vi "disk_setTemplateTail.vi"(8 "error in (no error)":errorcluster, 11 "Excel refnum":T1) -> (0 "error out":errorcluster, 2 "template tail":string[](array[string]), 3 "Excel refnum out":T1)   [LabVIEW 2017, in "NI_ExcelFile.lvlib"]
uses:
  <vilib>/express/express shared/NI_ExcelFile/NI_ExcelFile.lvlib
  <vilib>/express/express shared/NI_ExcelFile/Ctrls/ExcelRefnum.ctl
  <vilib>/express/express shared/NI_ExcelFile/Ctrls/MainData.ctl
  <vilib>/express/express shared/NI_ExcelFile/Ctrls/StreamMode.ctl
  <vilib>/express/express shared/NI_ExcelFile/Ctrls/TimeColumnMode.ctl
  <vilib>/express/express shared/NI_ExcelFile/Ctrls/FileAttribute.ctl
  <vilib>/express/express shared/NI_ExcelFile/Ctrls/Columns.ctl
  <vilib>/express/express shared/NI_ExcelFile/Ctrls/ColumnInfo.ctl
  <vilib>/express/express shared/NI_ExcelFile/Ctrls/DataType.ctl
  <vilib>/express/express shared/NI_ExcelFile/Ctrls/wd_recordInfo.ctl
  <vilib>/express/express shared/NI_ExcelFile/Ctrls/disk_TemplateFile.ctl
  <vilib>/express/express shared/NI_ExcelFile/Ctrls/meta_file.ctl
  <vilib>/express/express shared/NI_ExcelFile/Ctrls/meta_Block.ctl
  <vilib>/express/express shared/NI_ExcelFile/Ctrls/meta_BlockType.ctl
  <vilib>/express/express shared/NI_ExcelFile/Ctrls/TemplateEnum.ctl
  <vilib>/express/express shared/NI_ExcelFile/SubVIs/fmt_getUTF-8Text.vi
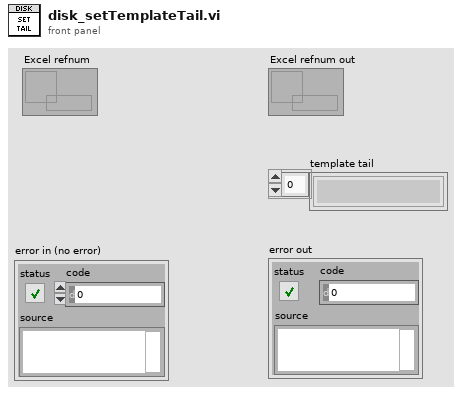
[diagram p1: front panel]
types:
  T1 = typedef "NI_ExcelFile.lvlib/ExcelRefnum.ctl" = refnum<data-value>
  T2 = typedef "NI_ExcelFile.lvlib/MainData.ctl" = cluster{"TargetFile":path, "StreamMode":T3, "Append?":bool, "ChunkSize":u64, "TimeColumnMode":T4, "TimestampFormat":string, "AbsoluteTime?":bool, "FileAttribute ":T5, "Column":T6, "FileRef":refnum<k1>, "MemoryRef":refnum<data-value>[], "RecordInfo":T9[], " ChannelPreviousInfo":u32[], "ChannelFirstRecord":u32[], "PredefinedFormattedValueLength":i64, "DiskTemplate":T10}
  T3 = typedef "NI_ExcelFile.lvlib/StreamMode.ctl" = enum16{"File", "Memory"}
  T4 = typedef "NI_ExcelFile.lvlib/TimeColumnMode.ctl" = enum16{"Empty", "OnePerCh", "One"}
  T5 = typedef "NI_ExcelFile.lvlib/FileAttribute.ctl" = cluster{"Creator":string, "Title":string, "SheetName":string}
  T6 = typedef "NI_ExcelFile.lvlib/Columns.ctl" = T7[]
  T7 = typedef "NI_ExcelFile.lvlib/ColumnInfo.ctl" = cluster{"Header":string, "Format":string, "DataType":T8, "Length":u64}
  T8 = typedef "NI_ExcelFile.lvlib/DataType.ctl" = enum16{"DDT", "WFM", "Array of STR", "Array of DBL", "Array of I8", "Array of I16", "Array of I32", "Array of I64", "Array of SGL", "Array of U8", "Array of U16", "Array of U32", "Array of U64", "Array of Time"}
  T9 = typedef "NI_ExcelFile.lvlib/wd_recordInfo.ctl" = cluster{"ChannelIndex":u32, "StartIndex":u64, "Length":u64, "Previous":i32, "Next":i32}
  T10 = typedef "NI_ExcelFile.lvlib/disk_TemplateFile.ctl" = cluster{"XMLRef":refnum<file>[], "ZipPath":path, "MetaFile":T11, "TempFolder":path}
  T11 = typedef "NI_ExcelFile.lvlib/meta_file.ctl" = cluster{"Ref":refnum<file>, "NextRow":i32, "NextPosition":i64, "Block":T12[]}
  T12 = typedef "NI_ExcelFile.lvlib/meta_Block.ctl" = cluster{"Version":u16, "Type":T13, "Length":i32, "Data":string}
  T13 = typedef "NI_ExcelFile.lvlib/meta_BlockType.ctl" = enum16{"NITag", "File", "Column"}
  T14 = typedef "NI_ExcelFile.lvlib/TemplateEnum.ctl" = enum16{"[Content_Types].xml", ".rels", "workbook.xml", "styles.xml", "workbook.xml.rels", "sheet.xml", "app.xml", "core.xml"}
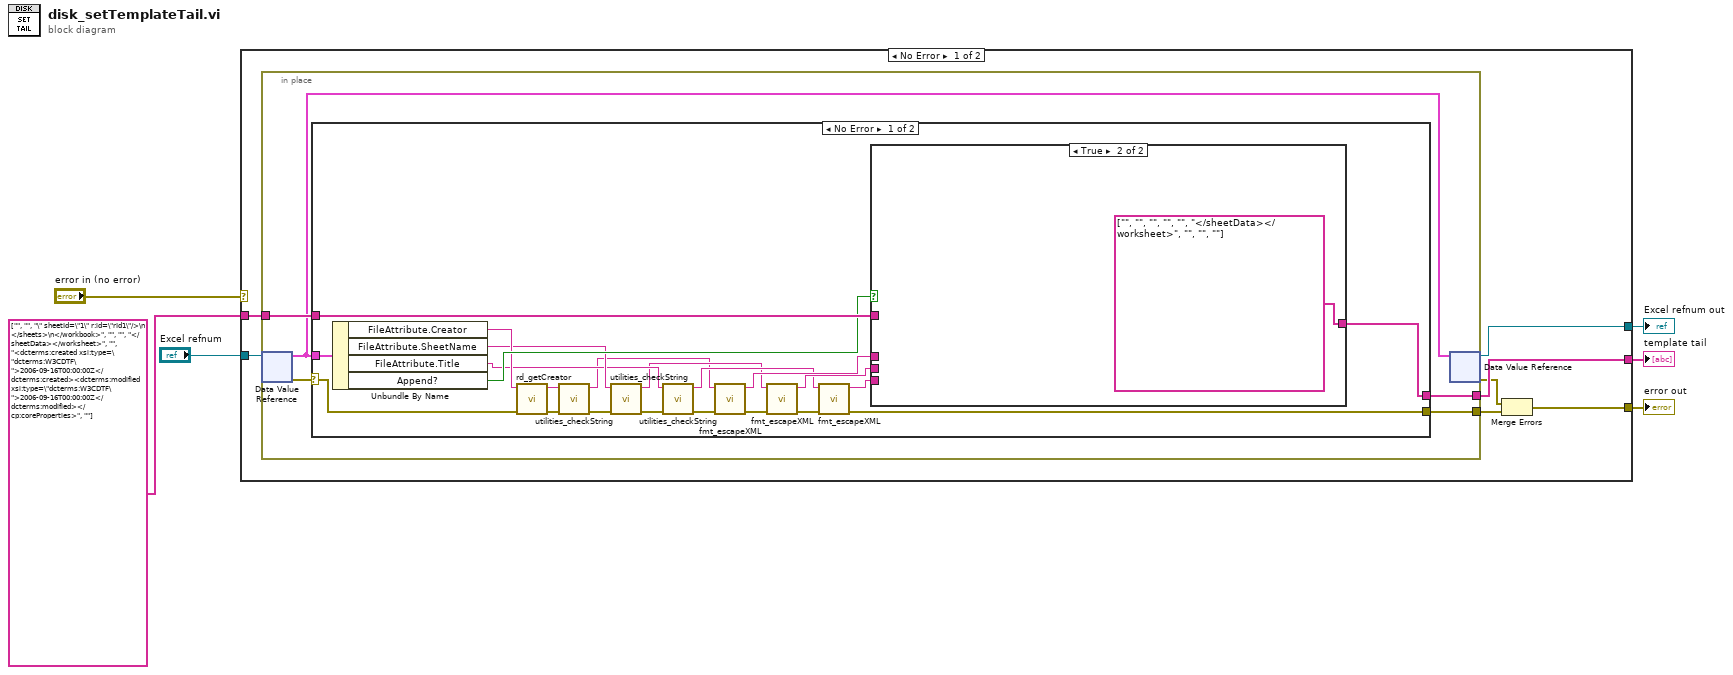
[diagram p0: block diagram]
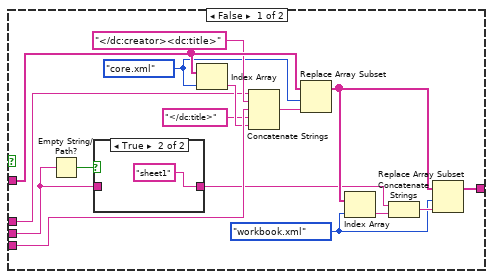
[diagram p2: hidden frame]
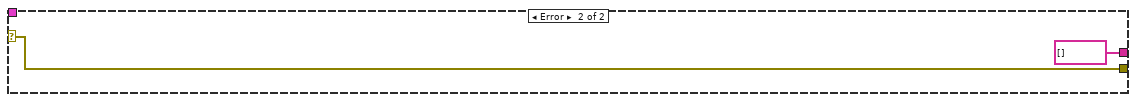
[diagram p4: hidden frame]
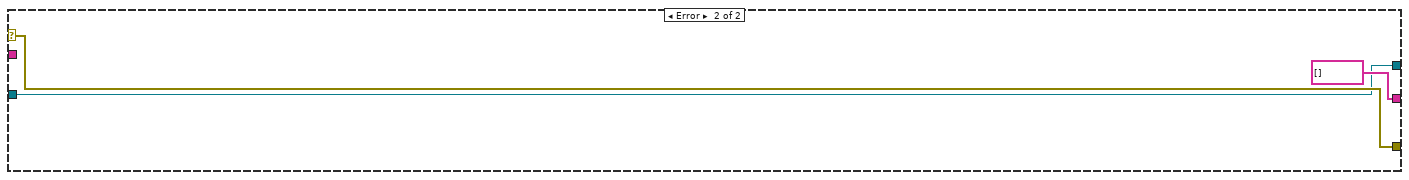
[diagram p5: hidden frame]
diagram:
  n1 = case shown="No Error" "error in (no error)" {
    selector: "error in (no error)" -> [_ w64]
    tunnel: string[] ["", "", "\" sheetId=\"1\" r:id=\"rId1\"/>\n  </sheets>\n</workbook>", "", "", "</sheetData></worksheet>", "", "<dcterms:created xsi:type=\"dcterms:W3CDTF\">2006-09-16T00:00:00Z</dcterms:created><dcterms:modified xsi:type=\"dcterms:W3CDTF\">2006-09-16T00:00:00Z</dcterms:modified></cp:coreProperties>", ""] -> [w13 _]
    tunnel: [w12 string[] []] -> w5
    tunnel: "Excel refnum" -> [w11 w62]
    tunnel: [w8 w64] -> w3
    tunnel: [w9 w62] -> w1
    frame No Error {
      n2 = in-place {
        in-place-border: w13 -> [w18]
        in-place-border: [w17] -> w12
        in-place-border: [w14] -> w7
        n3 = in-place-dvr #1(w11) -> (w16:T2, w15:errorcluster)
        n4 = case shown="No Error" w15 {
          selector: w15 -> [w32 w60]
          tunnel: w18 -> [w40 _]
          tunnel: [w39 string[] []] -> w17
          tunnel: w16 -> [w33 _]
          tunnel: [w29 w60] -> w14
          frame No Error {
            n5 = Unbundle By Name(w33) -> ("FileAttribute.Creator"=w34:string, "FileAttribute.SheetName"=w25:string, "FileAttribute.Title"=w23:string, "Append?"=w38:bool)
            n6 = call <vilib>:"rd_getCreator.vi"("error in (no error)"=w32, "creator"=w34) -> ("error out"=w27:errorcluster, "creator out"=w28:string)  [unwired: 8 in]
            n7 = call <vilib>:"utilities_checkString.vi"("error in (no error)"=w27, "String"=w28) -> ("error out"=w26:errorcluster, "String out"=w20:string)  [unwired: 8 in]
            n8 = call <vilib>:"utilities_checkString.vi"("error in (no error)"=w26, "String"=w25) -> ("error out"=w24:errorcluster, "String out"=w21:string)  [unwired: 8 in]
            n9 = call <vilib>:"utilities_checkString.vi"("error in (no error)"=w24, "String"=w23) -> ("error out"=w19:errorcluster, "String out"=w22:string)  [unwired: 8 in]
            n10 = call <vilib>:"fmt_escapeXML.vi"("error in"=w19, "plain text"=w20) -> ("error out"=w31:errorcluster, "xml text"=w37:string)  [unwired: 8 in]
            n11 = call <vilib>:"fmt_escapeXML.vi"("error in"=w31, "plain text"=w21) -> ("error out"=w30:errorcluster, "xml text"=w35:string)  [unwired: 8 in]
            n12 = call <vilib>:"fmt_escapeXML.vi"("error in"=w30, "plain text"=w22) -> ("error out"=w29:errorcluster, "xml text"=w36:string)  [unwired: 8 in]
            n13 = case shown="True" w38 {
              tunnel: w40 -> [w56 _]
              tunnel: [w52 string[] ["", "", "", "", "", "</sheetData></worksheet>", "", "", ""]] -> w39
              tunnel: w36 -> [w50 _]
              tunnel: w35 -> [w48 _]
              tunnel: w37 -> [w43 _]
              frame False {
                w41 = TemplateEnum."workbook.xml" ("Template")
                w42 = TemplateEnum."core.xml" ("Template")
                n14 = Empty String/Path?(string/path=w48) -> (empty?=w49:bool)
                n15 = case shown="True" w49 {
                  tunnel: [w57 "sheet1" ("string")] -> w44
                  tunnel: w48 -> [w57 _]
                  frame False {
                  }
                  frame True {
                  }
                }
                n16 = Index Array(array=w56, index=w42) -> (element=w47:string)
                n17 = Concatenate Strings(w43, "</dc:creator><dc:title>" ("string"), w50, "</dc:title>" ("string"), w47) -> (w45:string)
                n18 = Replace Array Subset(array=w56, new element=w45, index=w42) -> (w53:string[])
                n19 = Index Array(array=w53, index=w41) -> (element=w55:string)
                n20 = Concatenate Strings(w44, w55) -> (w54:string)
                n21 = Replace Array Subset(array=w53, new element=w54, index=w41) -> (w52:string[])
              }
              frame True {
              }
            }
          }
          frame Error {
          }
        }
        n22 = in-place-dvr #1(w16) -> (w9:T1, w10:errorcluster)
      }
      n23 = Merge Errors(w10, w7) -> (w8:errorcluster)
    }
    frame Error {
    }
  }
  "template tail" <- w5
  "error out" <- w3
  "Excel refnum out" <- w1
